vi "Display.vi"(8 "error in":errorcluster, 11 "Input (I32) in":refnum<class "Gif - Input (I32).lvclass">) -> (0 "error out":errorcluster, 3 "Input (I32) out":refnum<class "Gif - Input (I32).lvclass">)   [LabVIEW 2021, in "Gif - Input (I32).lvclass"]
doc: "This vi will display the input pop up waiting for a type I32 input from the user and will show a customized image.\n\n<b>Code Developed By:</b>\nDaniel Coons\nTechnology Service Corporation\n1983 S Liberty Drive\nBloomington, IN 47403\nPhone: 812 558-7100\ndaniel.coons@tsc.com\nwww.tsc.com/atcs"
uses:
  Gif - Input (I32).lvclass
  C:/Program Files/National Instruments/LabVIEW 2024/vi.lib/addons/_TSC/TSC Pop-Up/Popup/Popup.lvclass
  C:/Development/tsc-pop-up-gif/GIF Parent.lvclass
  Gif - Input (I32).lvclass/Gif - Input (I32).ctl
  <vilib>/addons/_TSC/TSC Pop-Up/Popup/Popup.lvclass/Popup.ctl
  GIF Parent.lvclass/GIF Parent.ctl
  <vilib>/addons/_TSC/TSC Pop-Up/Popup/Data Member Access/Read Theme.vi
  Read Delays.vi
  Read Gif Images.vi
  <vilib>/addons/_TSC/TSC Pop-Up/Theme/Theme.lvclass
  <vilib>/addons/_TSC/TSC Pop-Up/Popup/Popup.lvclass
  user32.dll
panel:
  in  "closer":bool
  out "header":bool
  in  "OK":bool
  in  "Input":i32
  out "Input value out":i32=1 min=1
  out "2D Picture":picture
  out "Message":string
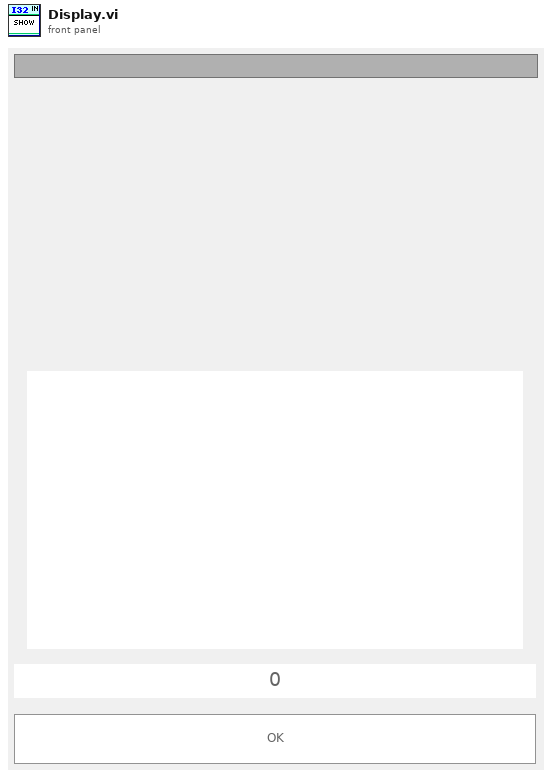
[diagram p1: front panel]
types:
  T1 = typedef "LVPoint32TypeDef.ctl" = cluster{"Horizontal":i32, "Vertical":i32}
  T2 = typedef "LVPositionTypeDef.ctl" = cluster{"Left":i32, "Top":i32}
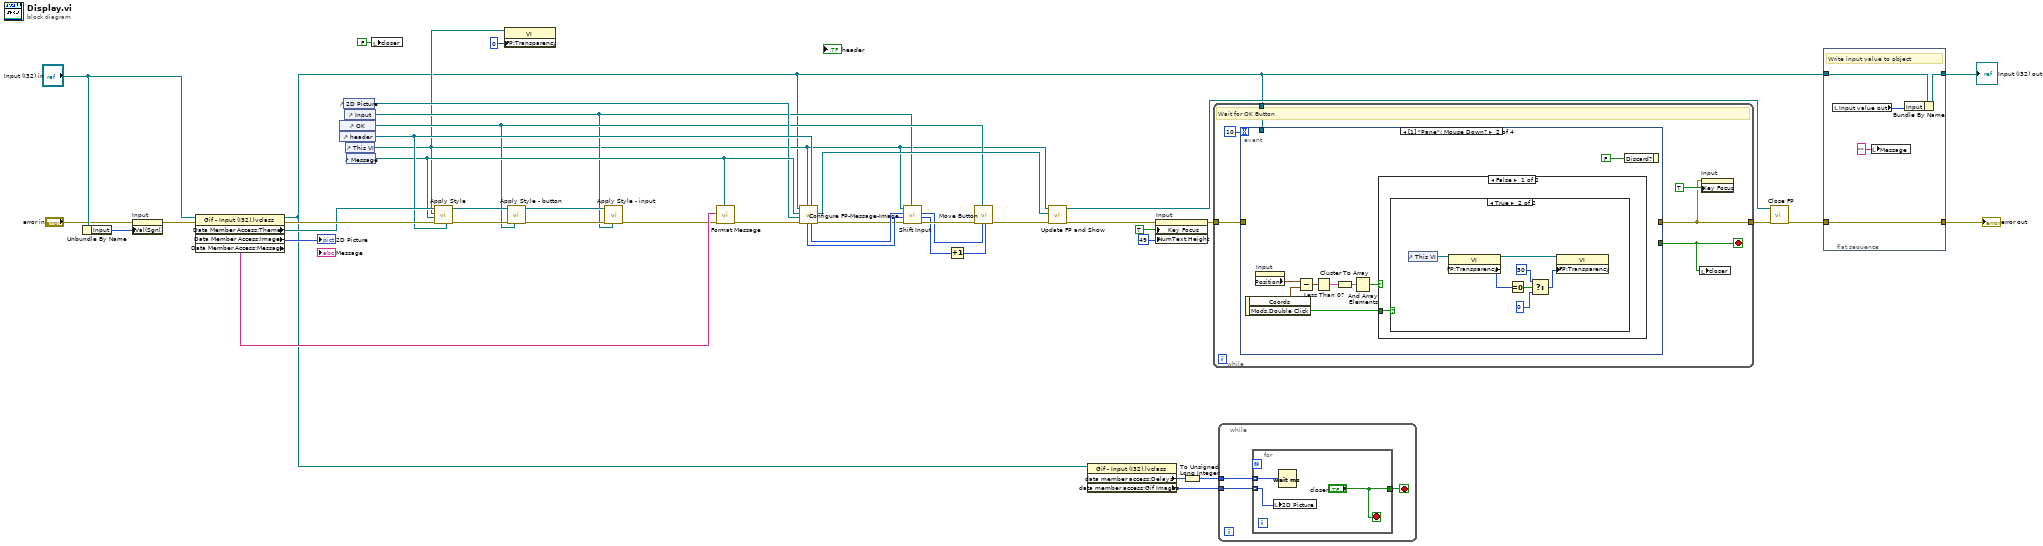
[diagram p0: block diagram]
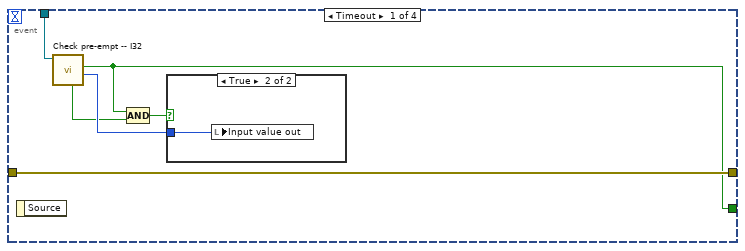
[diagram p2: hidden frame]
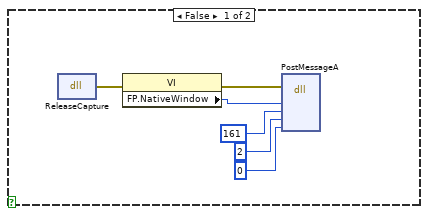
[diagram p4: hidden frame]
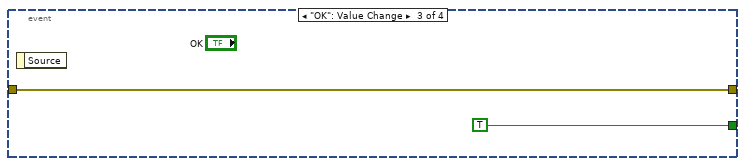
[diagram p6: hidden frame]
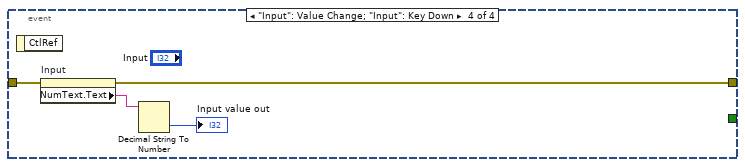
[diagram p7: hidden frame]
diagram:
  n1 = Unbundle By Name("Input (I32) in") -> ("Input"=w39:i32)
  n2 = property on="Input" class="DigNum (strict)"(error in="error in", "Val(Sgnl)"=w39) -> (error out=w40:errorcluster)  [unwired: 1 in, 1 out]
  n3 = property class="Gif - Input (I32).lvclass"(reference="Input (I32) in", error in=w40) -> (reference out=w1:refnum<class "Gif - Input (I32).lvclass">, error out=w38:errorcluster, "Data Member Access:Theme"=w28:refnum<class "Theme.lvclass">, "Data Member Access:Image"=→"2D Picture":picture, "Data Member Access:Message"=w30:string)
  n4 = control-ref of="OK"() -> (w11:refnum<vi>)
  n5 = control-ref of="header"() -> (w23:refnum<vi>)
  n6 = control-ref of="2D Picture"() -> (w21:refnum<vi>)
  n7 = control-ref of="Input"() -> (w10:refnum<vi>)
  n8 = control-ref of="This VI"() -> (w6:refnum<vi>)
  n9 = control-ref of="Message"() -> (w22:refnum<vi>)
  n10 = local write "closer"(FALSE ("closer")) -> ()
  n11 = call <vilib>:"Apply Style.vi"("header ref"=w23, "error in (no error)"=w38, "message ref"=w22, "pop up ref"=w6, "Theme in"=w28) -> ("error out"=w29:errorcluster, "Theme out"=w25:refnum<class "Theme.lvclass">)  [unwired: 5 in]
  n12 = property on="Property Node" class="VI"(reference=w6, "FP:Transparency"=u8 0 ("Front Panel Window:Transparency")) -> ()  [unwired: 1 in, 2 out]
  n13 = call <vilib>:"Apply Style - button.vi"("button ref"=w11, "error in (no error)"=w29, "Theme in"=w25) -> ("error out"=w27:errorcluster, "Theme out"=w24:refnum<class "Theme.lvclass">)  [unwired: 7 in]
  n14 = call <vilib>:"Apply Style - input.vi"("input ref"=w10, "error in (no error)"=w27, "Theme in"=w24) -> ("error out"=w26:errorcluster)  [unwired: 7 in, 1 out]
  n15 = call <vilib>:"Format Message.vi"("formatted string"=w22, "error in"=w26, "String Input"=w30) -> ("error out"=w31:errorcluster)  [unwired: 7 in, 1 out]
  n16 = call <vilib>:"Configure FP-Message-Image.vi"("header ref"=w23, "Pop Up ref"=w6, "error in (no error)"=w31, "Image ref"=w21, "Message ref"=w22, "Popup in"=w1) -> ("error out"=w13:errorcluster, "Panel Ref"=w12:refnum<vi>, "Panel Width"=w15:i32, "Panel Height"=w14:i32)  [unwired: 1 in, 1 out]
  n17 = call <vilib>:"Shift Input.vi"("Control"=w10, "Error In"=w13, "Panel Height"=w14, "Panel Width"=w15, "Pop Up ref"=w6) -> ("Error Out"=w20:errorcluster, "Panel Height out"=w18:i32, "Panel Width out"=w19:i32)  [unwired: 4 in]
  n18 = Increment(x=w18) -> (x+1=w17:i32)
  n19 = call <vilib>:"Move Button.vi"("Panel Height"=w17, "Panel Width"=w19, "Button"=w11, "Error In"=w20) -> ("Error Out"=w16:errorcluster)  [unwired: 6 in, 1 out]
  n20 = call <vilib>:"Update FP and Show.vi"("error in (no error)"=w16, "Panel Ref"=w12, "VI in"=w6) -> ("error out"=w35:errorcluster, "VI out"=w9:refnum<vi>)  [unwired: 7 in]
  n21 = property class="Gif - Input (I32).lvclass"(reference=w1) -> ("data member access:Delays"=w5:i32[], "data member access:Gif Images"=w4:picture[])  [unwired: 1 in, 2 out]
  n22 = property on="Input" class="DigNum (strict)"(error in=w35, "Key Focus"=TRUE, "NumText.Height"=u32 49 ("Numeric Text.Size:Height")) -> (error out=w34:errorcluster)  [unwired: 1 in, 1 out]
  n23 = To Unsigned Long Integer(number=w5) -> (unsigned 32bit integer=w3:u32[])
  n24 = while {
    tunnel: w34 -> [w50]
    tunnel: [w46] -> w37
    tunnel: w1 -> [w48]
    stop <- w45 stop-if-true
    # "Wait for OK Button"
    n25 = event shown="[1] \"Pane\": Mouse Down?" {
      selector: _ -> [_ _ _ _]
      dyn-events: _ -> [_ _ _ _]
      timeout: 10 -> [_ _ _ _]
      tunnel: w50 -> [w53 _ w81 w85]
      tunnel: [w53 _ w81 w83] -> w46
      tunnel: [w52 _ TRUE _] -> w45
      tunnel: w48 -> [w51 _ _ _]
      event Timeout {
        n26 = event-data() -> ()  [unwired: 1 in, 1 out]
        n27 = call <vilib>:"Check pre-empt -- I32.vi"("_Popup in"=w51) -> ("Value?"=w56:i32, "Pre-empted?"=w52:bool, "Type Match?"=w54:bool)  [unwired: 7 in, 1 out]
        n28 = Compound Arithmetic op=AND(w52, w54) -> (w55:bool)
        n29 = case shown="True" w55 {
          tunnel: w56 -> [_ w57]
          frame False {
          }
          frame True {
            n30 = local write "Input value out"(w57) -> ()
          }
        }
      }
      event Mouse Down? {
        n31 = event-data() -> ("Coords"=w59:T1, "Mods.Double Click"=w58:bool)  [unwired: 1 in]
        n32 = property on="Input" class="DigNum (strict)"() -> ("Position"=w60:T2)  [unwired: 2 in, 2 out]
        n33 = Subtract(x=w60, y=w59) -> (x-y=w61:T2)
        n34 = Less Than 0?(x=w61) -> (x < 0?=w62:cluster{"Left":bool, "Top":bool})
        n35 = Cluster To Array(cluster=w62) -> (array=w63:bool[])
        n36 = And Array Elements(Boolean array=w63) -> (logical AND=w64:bool)
        n37 = case shown="False" w64 {
          tunnel: w58 -> [w66 _]
          frame False {
            n38 = case shown="True" w66 {
              frame False {
                n39 = dll-call lib="user32.dll" fn="ReleaseCapture"() -> (error out=w70:errorcluster)  [unwired: 4 in, 1 out]
                n40 = property class="VI"(error in=w70) -> (error out=w71:errorcluster, "FP.NativeWindow"=w72:u64)  [unwired: 1 in, 1 out]
                n41 = dll-call lib="user32.dll" fn="PostMessageA"(error in=w71, "hWnd"=w72, "Msg"=161, "wParam"=2, "lParam"=0) -> ()  [unwired: 7 in, 2 out]
              }
              frame True {
                n42 = control-ref of="This VI"() -> (w79:refnum<vi>)
                n43 = property class="VI"(reference=w79) -> (reference out=w77:refnum<vi>, "FP:Transparency"=w78:u8)  [unwired: 1 in, 1 out]
                n44 = Equal To 0?(x=w78) -> (x = 0?=w76:bool)
                n45 = Select(t=u8 50, s=w76, f=u8 0) -> (s? t:f=w75:u8)
                n46 = property class="VI"(reference=w77, "FP:Transparency"=w75) -> ()  [unwired: 1 in, 2 out]
              }
            }
          }
          frame True {
          }
        }
        n47 = event-data("Discard?"=FALSE) -> ()  [unwired: 1 in, 1 out]
      }
      event "OK": Value Change {
        n48 = event-data() -> ()  [unwired: 1 in, 1 out]
      }
      event "Input": Value Change; "Input": Key Down {
        n49 = event-data() -> ()  [unwired: 1 in, 1 out]
        n50 = property on="Input" class="DigNum (strict)"(error in=w85) -> (error out=w83:errorcluster, "NumText.Text"=w84:string)  [unwired: 1 in, 1 out]
        n51 = Decimal String To Number(string=w84) -> (number=→"Input value out":i32)  [unwired: 2 in, 1 out]
      }
    }
    n52 = local write "closer"(w45) -> ()
    n53 = property on="Input" class="DigNum (strict)"(error in=w46, "Key Focus"=TRUE) -> ()  [unwired: 1 in, 2 out]
  }
  n54 = while {
    tunnel: w3 -> [w87]
    tunnel: w4 -> [w86]
    stop <- w88 stop-if-true
    n55 = for {
      tunnel: ["closer"] -> w88
      tunnel: w87 -> [w90] mode=indexing
      tunnel: w86 -> [w89] mode=indexing
      stop <- "closer" stop-if-true
      n56 = local write "2D Picture"(w89) -> ()
      n57 = Wait (ms)(milliseconds to wait=w90) -> ()  [unwired: 1 out]
    }
  }
  n58 = call <vilib>:"Close FP.vi"("error in (no error)"=w37, "VI in"=w9) -> ("error out"=w36:errorcluster)  [unwired: 9 in]
  n59 = flat-sequence {
    tunnel: w36 -> [w96]
    tunnel: [w96] -> w41
    tunnel: w1 -> [w95]
    tunnel: [w94] -> w42
    frame #0 {
      # "Write input value to object"
      n60 = local read "Input value out"() -> (w93:i32)
      n61 = local write "Message"("" ("Message")) -> ()
      n62 = Bundle By Name(cluster=w95, "Input"=w93) -> (w94:refnum<class "Gif - Input (I32).lvclass">)
    }
  }
  "error out" <- w41
  "Input (I32) out" <- w42
